vi "Generate Report as INI Section.vi"(7 "Parameters":variant, 8 "error in (no error)":errorcluster, 9 "Results":variant, 10 "Refnum in":T2, 11 "Analyze q-Factor in":refnum<class "Analyze q-Factor.lvclass">) -> (0 "error out":errorcluster, 2 "Refnum out":T2, 3 "Analyze q-Factor out":refnum<class "Analyze q-Factor.lvclass">)   [LabVIEW 2020, in "Analyze.lvlib" / "Analyze q-Factor.lvclass"]
uses:
  Analyze q-Factor.lvclass
  <vilib>/Utility/config.llb/Config Data RefNum.ctl
  Width Method.ctl
  <vilib>/Utility/config.llb/Write Key (String).vi
  <vilib>/Utility/config.llb/Write Key (Double).vi
  <vilib>/Utility/config.llb/NI_LVConfig.lvlib
panel:
  in  "Method":T1
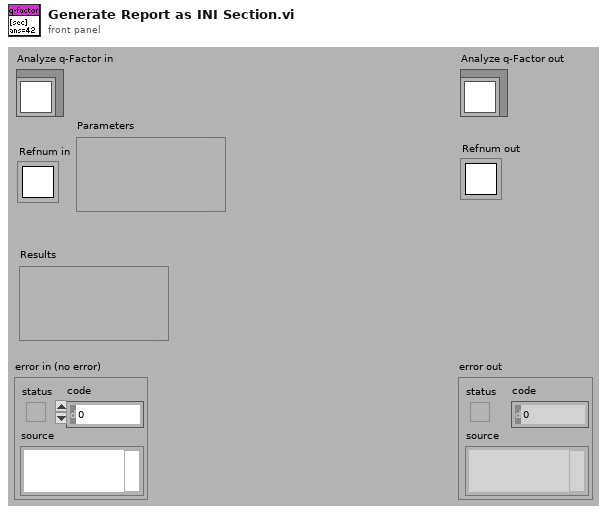
[diagram p1: front panel]
types:
  T1 = typedef "Width Method.ctl" = enum16{"FWHM", "1/e", "1/e^2", "80%", "90%"}
  T2 = typedef "NI_LVConfig.lvlib/Config Data RefNum.ctl" = refnum<k1>
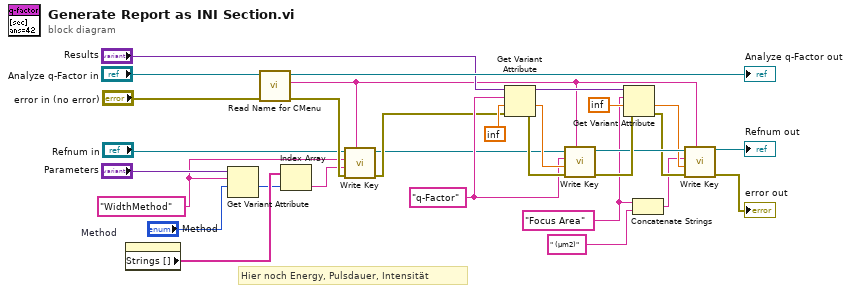
[diagram p0: block diagram]
diagram:
  w5 = "Focus Area" ("name")
  w14 = "WidthMethod" ("name")
  w17 = "q-Factor" ("name")
  # "Hier noch Energy, Pulsdauer, Intensität"
  n1 = property on="Method" class="Enum (strict)"() -> ("Strings []"=w19:string[])  [unwired: 2 in, 2 out]
  n2 = Get Variant Attribute(Variant="Parameters", name=w14, default value (empty Variant)="Method") -> (value=w18:T1)  [unwired: 1 in, 3 out]
  n3 = call-dynamic "Read Name for CMenu.vi"("error in (no error)"="error in (no error)", "Analyze BaseClass in"="Analyze q-Factor in") -> ("error out"=w16:errorcluster, "Name for Context menu"=w9:string, "Analyze BaseClass out"=→"Analyze q-Factor out":refnum<class "Analyze q-Factor.lvclass">)  [unwired: 7 in]
  n4 = Index Array(array=w19, index=w18) -> (element=w13:string)
  n5 = call-poly <vilib>:"Write Key.vi"("section"=w9, "error in (no error)"=w16, "value"=w13, "key"=w14, "refnum"="Refnum in") -> ("error out"=w15:errorcluster, "refnum out"=w1:T2)  [unwired: 4 in, 1 out]
  n6 = Get Variant Attribute(Variant="Results", name=w17, default value (empty Variant)=inf, error in=w15) -> (duplicate Variant=w22:variant, value=w25:dbl, error out=w24:errorcluster)  [unwired: 1 out]
  n7 = call-poly <vilib>:"Write Key.vi"("section"=w9, "error in (no error)"=w24, "value"=w25, "key"=w17, "refnum"=w1) -> ("error out"=w23:errorcluster, "refnum out"=w10:T2)  [unwired: 4 in, 1 out]
  n8 = Get Variant Attribute(Variant=w22, name=w5, default value (empty Variant)=inf, error in=w23) -> (value=w8:dbl, error out=w7:errorcluster)  [unwired: 2 out]
  n9 = Concatenate Strings(w5, " (µm2)" ("string")) -> (w6:string)
  n10 = call-poly <vilib>:"Write Key.vi"("section"=w9, "error in (no error)"=w7, "value"=w8, "key"=w6, "refnum"=w10) -> ("error out"=→"error out":errorcluster, "refnum out"=→"Refnum out":T2)  [unwired: 4 in, 1 out]
